vi "Stamp interface with PWM and calibration.vi"(8 "error in":errorcluster, 9 "sensor range error":bool, 10 "Plant State":u16(ring)=1) -> (0 "error out":errorcluster, 1 "NI board success":bool, 2 "Variables":cluster{string, "value":dbl}[](array[cluster]), 3 "Controls out 1":T1 {"fractional duty" format="%#_3g"})   [LabVIEW 2019]
uses:
  Process Controller 3.0/switch and fraction.ctl
  Process Controller 3.0/logic buffer cmd.ctl
  stamp command.ctl
panel:
  in  "Controls default":T1=[{"switch"=FALSE, "fractional duty"=0.0}, {"switch"=FALSE, "fractional duty"=0.0}, {"switch"=FALSE, "fractional duty"=0.0}, {"switch"=FALSE, "fractional duty"=0.0}, {"switch"=FALSE, "fractional duty"=0.0}, {"switch"=FALSE, "fractional duty"=0.0}, {"switch"=FALSE, "fractional duty"=0.0}, {"switch"=FALSE, "fractional duty"=0.0}, {"switch"=FALSE, "fractional duty"=0.0}, {"switch"=FALSE, "fractional duty"=0.0}, {"switch"=FALSE, "fractional duty"=0.0}, {"switch"=FALSE, "fractional duty"=0.0}, {"switch"=FALSE, "fractional duty"=0.0}, {"switch"=FALSE, "fractional duty"=0.0}, {"switch"=FALSE, "fractional duty"=0.0}, {"switch"=FALSE, "fractional duty"=0.0}] {"fractional duty" format="%#_3g"}
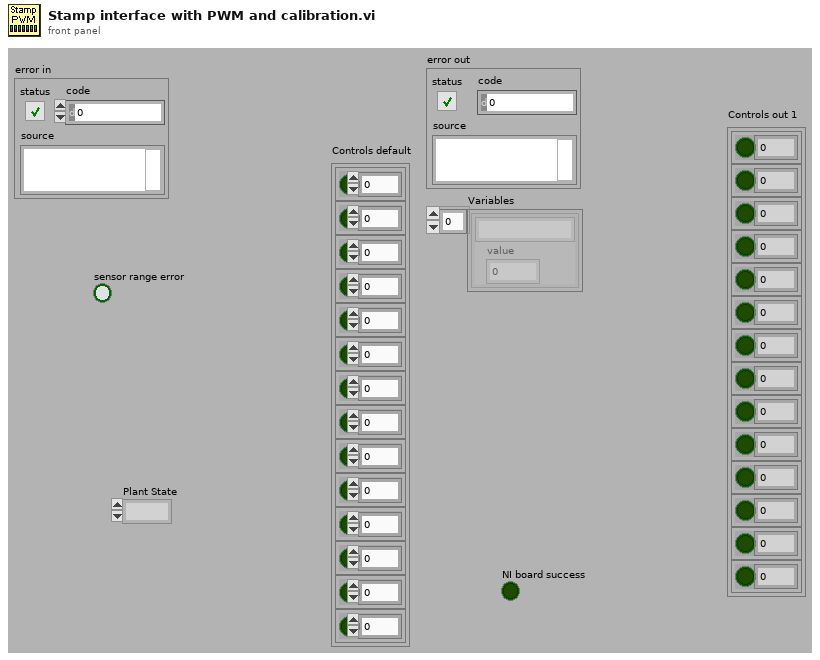
[diagram p1: front panel]
types:
  T1 = typedef "switch and fraction.ctl" = cluster{"switch":bool, "fractional duty":dbl}[]
  T2 = typedef "logic buffer cmd.ctl" = enum16{"read", "write ouput settings", "write rules", "write setpoints", "write output descriptions", "write all", "calculate setpoints", "save", "open", "Load all setpoint code", "Load one setpoint code", "Configure one setpoint code"}
  T3 = typedef "stamp command.ctl" = enum16{"Configure", "Write", "Off", "Close"}
  T4 = typedef "variable setpoint.ctl" = cluster{"name":string, "unit":string, "value":dbl, "Type":enum16{"Constant", "Variable"}, "variable":cluster{"selected sensors":i32[], "selected set points":i32[], "VI":path, "Data average interval":T5, "code ref":T6}}
  T5 = typedef "data ave interval.ctl" = dbl
  T6 = typedef "type specifier for control code.ctl" = refnum<vi>
  T7 = typedef "Output control.ctl" = u16[][]
  T8 = typedef "Stamp 2 control.ctl" = cluster{"Switches":bool[], "Pumps":T9[]}
  T9 = typedef "Pump w direction.ctl" = cluster{"on/off":T10, "Direction":T11, "flow rate":dbl[unit], "Tubing":T12, "tubing or 0 to 1":bool, "0 to 1":dbl}
  T10 = typedef "mini peristaltic pump.ctl" = bool
  T11 = typedef "Pump Direction.ctl" = bool
  T12 = typedef "3-stop colors and numbers.ctl" = enum16{"orange-black", "orange-red", "orange-blue", "orange-green", "green-yellow", "orange-yellow", "white-yellow", "orange-white", "black-black", "orange-orange", "white-black", "white-white", "white-red", "red-red", "red-grey", "grey-grey", "yellow-yellow", "yellow-blue", "blue-blue", "blue-green", "green-green", "purple-purple", "purple-black", "purple-orange", "purple-white", "black-white", "13", "14", "15", "16", "17", "18"}
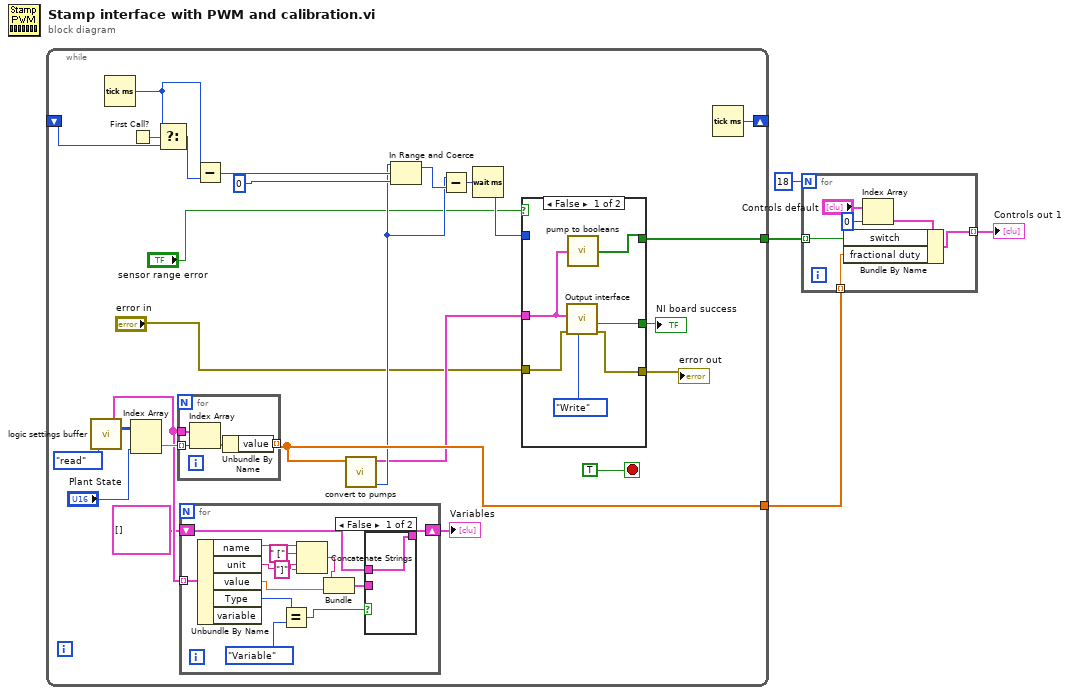
[diagram p0: block diagram]
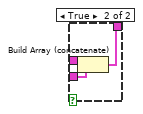
[diagram p2: hidden frame]
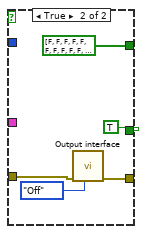
[diagram p3: hidden frame]
diagram:
  n1 = while {
    shift-right: [w21] -> _
    shift-left: _ -> [w26]
    tunnel: [w13] -> w4
    tunnel: [w19] -> w2
    stop <- TRUE stop-if-true
    n2 = call "logic settings buffer.vi"("command"=logic_buffer_cmd."read") -> ("Set Points out"=w7:T4[], "ouput settings out"=w29:T7)  [unwired: 11 in, 6 out]
    n3 = Tick Count (ms)() -> (millisecond timer value=w20:u32)
    n4 = First Call?() -> (First Call?: T/F=w27:bool)
    n5 = Index Array(array=w29, index (col)="Plant State") -> (element=w17:u16[])  [unwired: 1 in]
    n6 = Select(t=w20, s=w27, f=w26) -> (s? t:f=w25:u32)
    n7 = for {
      tunnel: w17 -> [w62] mode=indexing
      tunnel: w7 -> [w61]
      tunnel: [w59] -> w13 mode=indexing
      n8 = Index Array(array=w61, index=w62) -> (element=w60:T4)
      n9 = Unbundle By Name(w60) -> ("value"=w59:dbl)
    }
    n10 = for {
      tunnel: w7 -> [w43] mode=indexing
      shift-right: [w39] -> w5
      shift-left: cluster{string, "value":dbl}[] [] -> [w40]
      n11 = Unbundle By Name(w43) -> ("name"=w36:string, "unit"=w34:string, "value"=w37:dbl, "Type"=w42:enum16{"Constant", "Variable"})  [unwired: 1 out]
      n12 = Equal?(x=w42, y=enum16{"Constant", "Variable"}."Variable" ("Type")) -> (x = y?=w31:bool)
      n13 = Concatenate Strings(w36, " [" ("string"), w34, "]" ("string")) -> (w32:string)
      n14 = Bundle(w32, "value"=w37) -> (w38:cluster{string, "value":dbl})  [unwired: 1 in]
      n15 = case shown="False" w31 {
        tunnel: w40 -> [w44 w47]
        tunnel: [w44 w46] -> w39
        tunnel: w38 -> [_ w45]
        frame False {
        }
        frame True {
          n16 = Build Array (concatenate)(w47, w45) -> (w46:cluster{string, "value":dbl}[])
        }
      }
    }
    "Variables" <- w5
    n17 = Subtract(x=w20, y=w25) -> (x-y=w24:u32)
    n18 = call "convert to pumps.vi"("control values"=w13) -> ("minimum pulse time (ms) 2"=w12:u32, "Control out"=w11:T8)  [unwired: 9 in]
    n19 = In Range and Coerce(upper limit=w12, x=w24, lower limit=u32 0) -> (coerced(x)=w22:u32)  [unwired: 1 out]
    n20 = Subtract(x=w12, y=w22) -> (x-y=w16:u32)
    n21 = Wait (ms)(milliseconds to wait=w16) -> (millisecond timer value=w15:u32)
    n22 = case shown="False" "sensor range error" {
      tunnel: [w51 bool[] [FALSE, FALSE, FALSE, FALSE, FALSE, FALSE, FALSE, FALSE, FALSE, FALSE, FALSE, FALSE, FALSE, FALSE, FALSE, FALSE, FALSE, FALSE, FALSE, FALSE, FALSE, FALSE, FALSE, FALSE, FALSE, FALSE, FALSE, FALSE, FALSE, FALSE, FALSE, FALSE] ("inverting")] -> w19
      tunnel: w15 -> [_ _]
      tunnel: [w52 TRUE ("success?")] -> w14
      tunnel: w11 -> [w50 _]
      tunnel: "error in" -> [w49 w55]
      tunnel: [w48 w54] -> w9
      frame False {
        n23 = call "Output interface.vi"("Stamp Command"=stamp_command."Write", "error in"=w49, "Control"=w50) -> ("error out"=w48:errorcluster, "success?"=w52:bool)  [unwired: 7 in]
        n24 = call "pump to booleans.vi"("Control"=w50) -> ("controls boolean"=w51:bool[])
      }
      frame True {
        n25 = call "Output interface.vi"("Stamp Command"=stamp_command."Off", "error in"=w55) -> ("error out"=w54:errorcluster)  [unwired: 8 in, 1 out]
      }
    }
    "NI board success" <- w14
    "error out" <- w9
    n26 = Tick Count (ms)() -> (millisecond timer value=w21:u32)
  }
  n27 = for {
    N: 18 -> [_]
    tunnel: w2 -> [w68] mode=indexing
    tunnel: w4 -> [w67] mode=indexing
    tunnel: [w66] -> w1 mode=indexing
    n28 = Index Array(array="Controls default", index=0) -> (element=w63:cluster{"switch":bool, "fractional duty":dbl})
    n29 = Bundle By Name(cluster=w63, "switch"=w68, "fractional duty"=w67) -> (w66:cluster{"switch":bool, "fractional duty":dbl})
  }
  "Controls out 1" <- w1
